vi "Weather Download App.vi"() -> ()   [LabVIEW 2012]
uses:
  TypeDef/Loop States.ctl
  TypeDef/WeatherData.ctl
  GUI Helpers/Status Helper Action.ctl
  <vilib>/addons/database/Connection.llb/Conn ObjectReference.ctl
  <vilib>/httpClient/ClientHandle.ctl
  <vilib>/addons/database/Connection.llb/DB Tools Open Connec (Path).vi
  <vilib>/httpClient/LabVIEWHTTPClient.lvlib
  <vilib>/addons/database/NI_Database_API.lvlib
panel:
  out "Push to DB error out":errorcluster
  out "# Data Lines in queue":i32
  out "Get Data error out":errorcluster
  out "Push To DB Loop State":T1
  out "Get Data Loop State":T1
  out "# Dates in queue":i32
  out "Push to DB":dbl(slide) scale=0.0..1.0
  out "Get Http Data":dbl(slide) scale=0.0..1.0
  out "Days in to Queue":dbl(slide) scale=0.0..1.0
  out "Days":i32
  in  "Abort":bool
  in  "Start":bool
  in  "DB Table Name":string="weatherdata"
  in  "DB Password":string="password123%%%"
  in  "DB Username":string="john"
  in  "DB Connection Information":path=path "D:/SVN/RHOK/WeatherDownloader/src/DB Interface/Crashbang.lisa.duffnet.local.udl"
  in  "Airport Code":string
  in  "End Time Stamp":timestamp format="%<%m/%d/%Y>T"
  in  "Start Time Stamp":timestamp format="%<%m/%d/%Y>T"
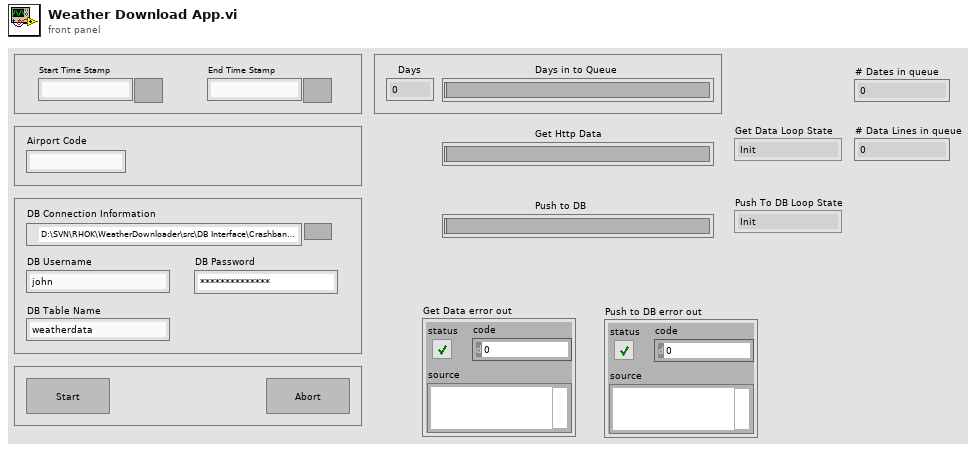
[diagram p1: front panel]
types:
  T1 = typedef "Loop States.ctl" = enum16{"Init", "Run Data", "Shutdown"}
  T2 = typedef "WeatherData.ctl" = cluster{"TimeEST":timestamp, "TemperatureF":dbl, "DewPointF":dbl, "Humidity":i32, "Sea Level PressureIn":dbl, "VisibilityMPH":dbl, "Wind Direction":string, "Wind SpeedMPH":dbl, "Gust SpeedMPH":dbl, "PrecipitationIn":dbl, "Events":string, "Conditions":string, "WindDirDegrees":i32, "datetimeest":timestamp}
  T3 = typedef "Status Helper Action.ctl" = enum16{"Init", "Load Number Of Days", "Inc Add to Queue ", "Inc Get HTTP Data", "Add Push to DB", "Inc Push To DB", "Read"}
  T4 = typedef "LabVIEWHTTPClient.lvlib/ClientHandle.ctl" = refnum<k1>
  T5 = typedef "NI_Database_API.lvlib/Conn ObjectReference.ctl" = refnum<k1>
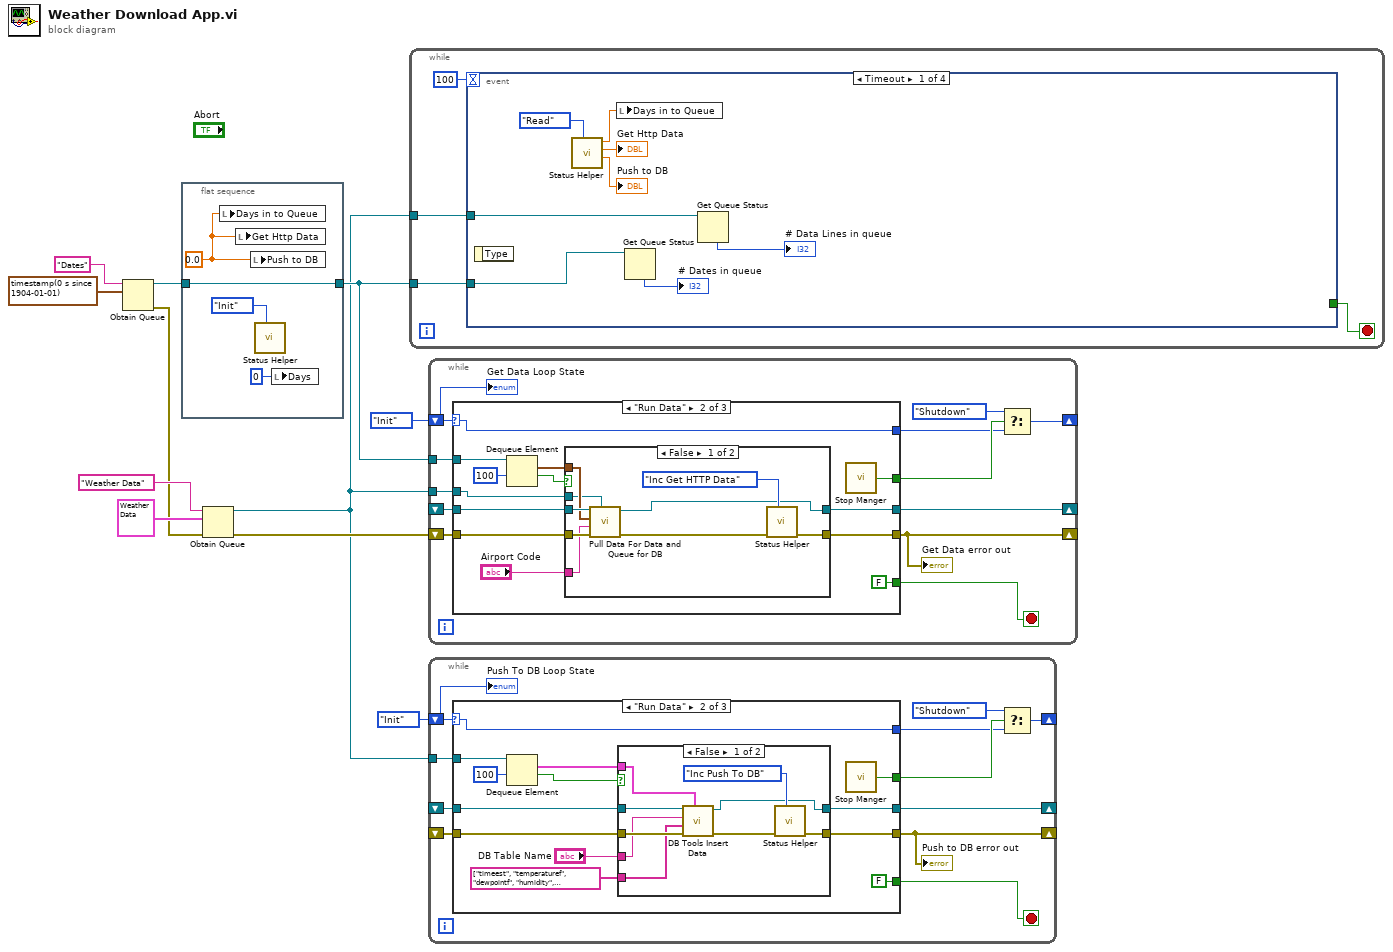
[diagram p0: block diagram]
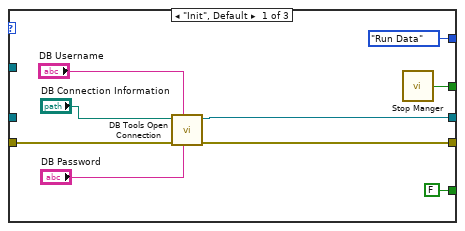
[diagram p2: hidden frame]
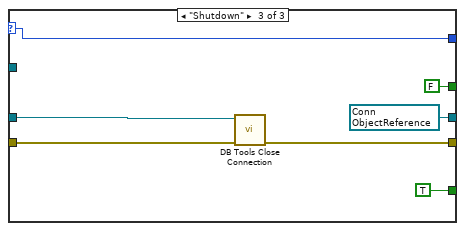
[diagram p4: hidden frame]
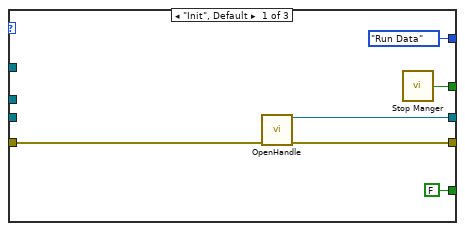
[diagram p5: hidden frame]
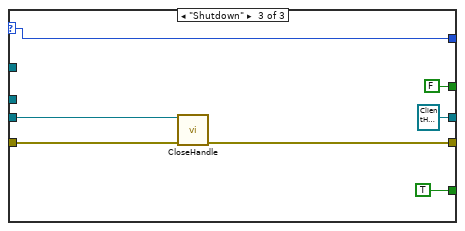
[diagram p7: hidden frame]
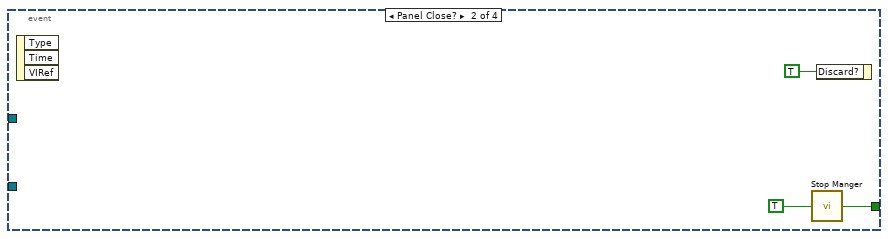
[diagram p8: hidden frame]
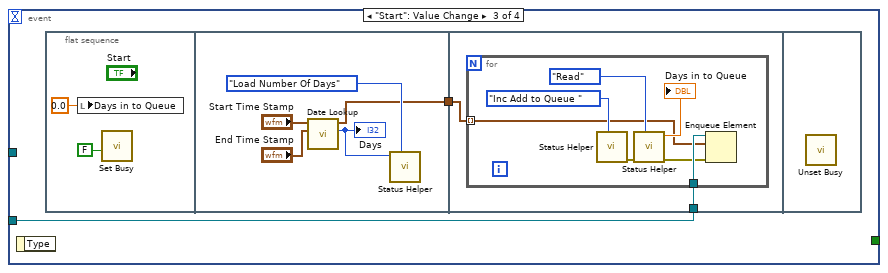
[diagram p9: hidden frame]
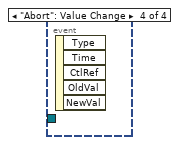
[diagram p10: hidden frame]
diagram:
  n1 = Obtain Queue(name (unnamed)="Dates", element data type=timestamp(0 s since 1904-01-01)) -> (queue out=w9:refnum<queue>, error out=w4:errorcluster)  [unwired: 3 in, 1 out]
  n2 = flat-sequence {
    tunnel: [w15] -> w8
    tunnel: w9 -> [w15]
    frame #0 {
      w14 = 0.0 ("Push to DB")
      n3 = local write "Days in to Queue"(w14) -> ()
      n4 = local write "Get Http Data"(w14) -> ()
      n5 = local write "Push to DB"(w14) -> ()
      n6 = call "Status Helper"("Action"=Status_Helper_Action."Init") -> ()  [unwired: 7 in, 4 out]
      n7 = local write "Days"(0 ("Days")) -> ()
    }
  }
  n8 = Obtain Queue(name (unnamed)="Weather Data", element data type=T2 {"TimeEST"=timestamp(0 s since 1904-01-01), "TemperatureF"=0.0, "DewPointF"=0.0, "Humidity"=0, "Sea Level PressureIn"=0.0, "VisibilityMPH"=0.0, "Wind Direction"="", "Wind SpeedMPH"=0.0, "Gust SpeedMPH"=0.0, "PrecipitationIn"=0.0, "Events"="", "Conditions"="", "WindDirDegrees"=0, "datetimeest"=timestamp(0 s since 1904-01-01)} ("weatherdata"), error in (no error)=w4) -> (queue out=w1:refnum<queue>, error out=w3:errorcluster)  [unwired: 2 in, 1 out]
  n9 = while {
    tunnel: w8 -> [w17]
    tunnel: w1 -> [w16]
    stop <- w18 stop-if-true
    n10 = event shown="[0] Timeout" {
      selector: _ -> [_ _ _ _]
      dyn-events: _ -> [_ _ _ _]
      timeout: 100 -> [_ _ _ _]
      tunnel: [_ w28 _ _] -> w18
      tunnel: w17 -> [w23 _ w31 _]
      tunnel: w16 -> [w21 _ _ _]
      event Timeout {
        n11 = event-data() -> ()  [unwired: 1 in, 1 out]
        n12 = call "Status Helper"("Action"=Status_Helper_Action."Read") -> ("% Push To DB"=→"Push to DB":dbl, "% Get Http Data"=→"Get Http Data":dbl, "% Add to QUEUE"=w27:dbl)  [unwired: 7 in, 1 out]
        n13 = local write "Days in to Queue"(w27) -> ()
        n14 = Get Queue Status(queue=w23) -> (# elements in queue=→"# Dates in queue":i32)  [unwired: 2 in, 7 out]
        n15 = Get Queue Status(queue=w21) -> (# elements in queue=→"# Data Lines in queue":i32)  [unwired: 2 in, 7 out]
      }
      event Panel Close? {
        n16 = event-data() -> ()  [unwired: 1 in, 3 out]
        n17 = call "Stop Manger.vi"("Stop (F)"=TRUE ("Discard?")) -> ("Loop Stop"=w28:bool)  [unwired: 1 in]
        n18 = event-data("Discard?"=TRUE) -> ()  [unwired: 1 in, 1 out]
      }
      event "Start": Value Change {
        n19 = event-data() -> ()  [unwired: 1 in, 1 out]
        n20 = flat-sequence {
          tunnel: [w35] -> w32
          tunnel: w32 -> [w41]
          tunnel: w31 -> [w40]
          frame #0 {
            n21 = local write "Days in to Queue"(0.0 ("Days in to Queue")) -> ()
            n22 = call <vilib>:"Set Busy.vi"("disable click? (T)"=FALSE) -> ()  [unwired: 9 in, 2 out]
          }
          frame #1 {
            n23 = call "Date Lookup.vi"("End Time Stamp"="End Time Stamp", "Start Time Stamp"="Start Time Stamp") -> ("Number of Days"=w37:i32, "DateTime Array"=w35:timestamp[])  [unwired: 8 in]
            "Days" <- w37
            n24 = call "Status Helper"("Action"=Status_Helper_Action."Load Number Of Days", "Number of Days"=w37) -> ()  [unwired: 6 in, 4 out]
          }
          frame #2 {
            n25 = for {
              tunnel: w41 -> [w42] mode=indexing
              tunnel: w40 -> [w44]
              n26 = call "Status Helper"("Action"=Status_Helper_Action."Inc Add to Queue ") -> ("error out"=w47:errorcluster)  [unwired: 7 in, 3 out]
              n27 = call "Status Helper"("Action"=Status_Helper_Action."Read", "error in (no error)"=w47) -> ("error out"=w43:errorcluster, "% Add to QUEUE"=→"Days in to Queue":dbl)  [unwired: 6 in, 2 out]
              n28 = Enqueue Element(queue=w44, element=w42, error in (no error)=w43) -> ()  [unwired: 1 in, 3 out]
            }
          }
          frame #3 {
            n29 = call <vilib>:"Unset Busy.vi"() -> ()  [unwired: 11 in, 1 out]
          }
        }
      }
      event "Abort": Value Change {
        n30 = event-data() -> ()  [unwired: 1 in, 5 out]
      }
    }
  }
  n31 = while {
    tunnel: w8 -> [w60]
    shift-right: [w55] -> _
    shift-left: Loop_States."Init" -> [w59]
    shift-right: [w52] -> _
    shift-left: w3 -> [w50]
    shift-right: [w53] -> _
    shift-left: _ -> [w51]
    tunnel: w1 -> [w49]
    stop <- w58 stop-if-true
    n32 = case shown="\"Run Data\"" w59 {
      selector: w59 -> [_ w70 w91]
      tunnel: w60 -> [_ w79 _]
      tunnel: [FALSE ("Loop Stop") FALSE ("Loop Stop") TRUE ("Loop Stop")] -> w58
      tunnel: [w66 w69 FALSE ("Loop Stop")] -> w57
      tunnel: [Loop_States."Run Data" w70 w91] -> w56
      tunnel: [w63 w72 T4 refnum ("client handle out")] -> w53
      tunnel: [w62 w73 w92] -> w52
      tunnel: w51 -> [_ w71 w94]
      tunnel: w50 -> [w61 w74 w93]
      tunnel: w49 -> [_ w68 _]
      frame "Init", Default {
        n33 = call <vilib>:"OpenHandle.vi"("error in (no error)"=w61) -> ("client handle out"=w63:T4, "error out"=w62:errorcluster)  [unwired: 13 in]
        n34 = call "Stop Manger.vi"() -> ("Loop Stop"=w66:bool)  [unwired: 2 in]
      }
      frame "Run Data" {
        n35 = Dequeue Element(queue=w79, timeout in ms (-1)=100) -> (element=w76:timestamp, timed out?=w77:bool)  [unwired: 1 in, 2 out]
        n36 = case shown="False" w77 {
          tunnel: w76 -> [w81 _]
          tunnel: w74 -> [w84 w90]
          tunnel: [w87 w90] -> w73
          tunnel: [w85 w89] -> w72
          tunnel: w71 -> [w86 w89]
          tunnel: w68 -> [w80 _]
          tunnel: "Airport Code" -> [w82 _]
          frame False {
            n37 = call "Pull Data For Data and Queue for DB.vi"("Weather Data queue"=w80, "error in (no error)"=w84, "Airport Code"=w82, "Time Stamp"=w81, "Refnum in"=w86) -> ("error out"=w83:errorcluster, "Refnum out"=w85:T4)  [unwired: 5 in]
            n38 = call "Status Helper"("Action"=Status_Helper_Action."Inc Get HTTP Data", "error in (no error)"=w83) -> ("error out"=w87:errorcluster)  [unwired: 6 in, 3 out]
          }
          frame True {
          }
        }
        n39 = call "Stop Manger.vi"() -> ("Loop Stop"=w69:bool)  [unwired: 2 in]
      }
      frame "Shutdown" {
        n40 = call <vilib>:"CloseHandle.vi"("client handle"=w94, "error in (no error)"=w93) -> ("error out"=w92:errorcluster)  [unwired: 13 in]
      }
    }
    "Get Data error out" <- w52
    n41 = Select(t=Loop_States."Shutdown", s=w57, f=w56) -> (s? t:f=w55:T1)
    "Get Data Loop State" <- w59
  }
  n42 = while {
    tunnel: w1 -> [w108]
    shift-right: [w103] -> _
    shift-left: Loop_States."Init" -> [w107]
    shift-right: [w98] -> _
    shift-left: _ -> [w99]
    shift-right: [w101] -> _
    shift-left: _ -> [w100]
    stop <- w106 stop-if-true
    n43 = case shown="\"Run Data\"" w107 {
      selector: w107 -> [_ w121 w146]
      tunnel: w108 -> [_ w130 _]
      tunnel: [FALSE ("Loop Stop") FALSE ("Loop Stop") TRUE ("Loop Stop")] -> w106
      tunnel: [w117 w120 FALSE ("Loop Stop")] -> w105
      tunnel: [Loop_States."Run Data" w121 w146] -> w104
      tunnel: [w114 w123 w142] -> w101
      tunnel: [w112 w124 w143] -> w98
      tunnel: w100 -> [_ w122 w145]
      tunnel: w99 -> [w113 w125 w144]
      frame "Init", Default {
        n44 = call-poly <vilib>:"DB Tools Open Connection.vi"("password"="DB Password", "userID"="DB Username", "error in (no error)"=w113, "connection information"="DB Connection Information") -> ("error out"=w112:errorcluster, "connection reference"=w114:T5)  [unwired: 4 in]
        n45 = call "Stop Manger.vi"() -> ("Loop Stop"=w117:bool)  [unwired: 2 in]
      }
      frame "Run Data" {
        n46 = Dequeue Element(queue=w130, timeout in ms (-1)=100) -> (element=w127:T2, timed out?=w128:bool)  [unwired: 1 in, 2 out]
        n47 = case shown="False" w128 {
          tunnel: w127 -> [w133 _]
          tunnel: w125 -> [w135 w141]
          tunnel: [w138 w141] -> w124
          tunnel: [w136 w140] -> w123
          tunnel: w122 -> [w137 w140]
          tunnel: "DB Table Name" -> [w132 _]
          tunnel: string[] ["timeest", "temperaturef", "dewpointf", "humidity", "sealevelpressurein", "visibilitymph", "winddirection", "windspeedmph", "gustspeedmph", "precipitationin", "events", "conditions", "winddirdegrees", "datetimeest"] ("subarray 3") -> [w131 _]
          frame False {
            n48 = call <vilib>:"DB Tools Insert Data.vi"("data"=w133, "error in (no error)"=w135, "columns"=w131, "table"=w132, "connection reference"=w137) -> ("error out"=w134:errorcluster, "connection reference out"=w136:T5)  [unwired: 5 in]
            n49 = call "Status Helper"("Action"=Status_Helper_Action."Inc Push To DB", "error in (no error)"=w134) -> ("error out"=w138:errorcluster)  [unwired: 6 in, 3 out]
          }
          frame True {
          }
        }
        n50 = call "Stop Manger.vi"() -> ("Loop Stop"=w120:bool)  [unwired: 2 in]
      }
      frame "Shutdown" {
        w142 = T5 refnum items=["Connection"] ("connection reference")
        n51 = call <vilib>:"DB Tools Close Connection.vi"("error in (no error)"=w144, "connection reference"=w145) -> ("error out"=w143:errorcluster)  [unwired: 5 in]
      }
    }
    "Push to DB error out" <- w98
    n52 = Select(t=Loop_States."Shutdown", s=w105, f=w104) -> (s? t:f=w103:T1)
    "Push To DB Loop State" <- w107
  }
